vi "Global Variables.vi"() -> ()   [LabVIEW 2019]
panel:
  in  "Motor":i32
  in  "Device Address":i32
  in  "Device Key":string
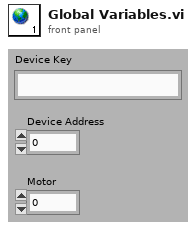
[diagram p1: front panel]
diagram:
